vi "文件名.vi"() -> (3 "保存文件名 2":string)   [LabVIEW 2017]
panel:
  in  "保存文件名":string
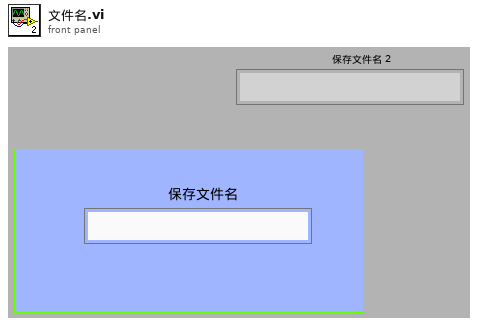
[diagram p1: front panel]
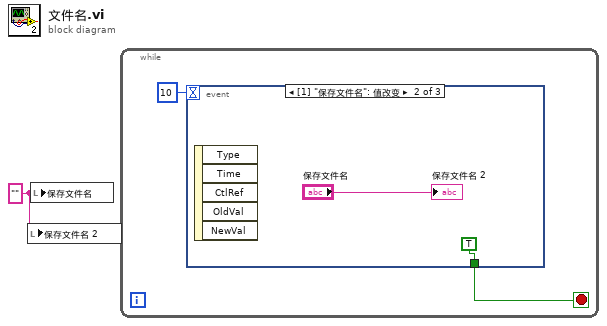
[diagram p0: block diagram]
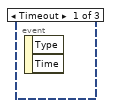
[diagram p2: hidden frame]
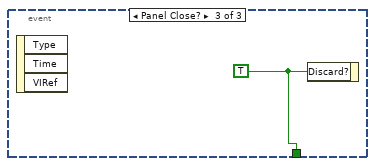
[diagram p3: hidden frame]
diagram:
  w1 = "" ("保存文件名")
  n1 = local write "保存文件名 2"(w1) -> ()
  n2 = local write "保存文件名"(w1) -> ()
  n3 = while {
    stop <- w2 stop-if-true
    n4 = event shown="[1] \"保存文件名\": 值改变" {
      selector: _ -> [_ _ _]
      dyn-events: _ -> [_ _ _]
      timeout: 10 -> [_ _ _]
      tunnel: [_ TRUE w6] -> w2
      event Timeout {
        n5 = event-data() -> ()  [unwired: 1 in, 2 out]
      }
      event "保存文件名": Value Change {
        n6 = event-data() -> ()  [unwired: 1 in, 5 out]
        "保存文件名 2" <- "保存文件名"
      }
      event Panel Close? {
        w6 = TRUE ("放弃？")
        n7 = event-data() -> ()  [unwired: 1 in, 3 out]
        n8 = event-data("Discard?"=w6) -> ()  [unwired: 1 in, 1 out]
      }
    }
  }
